vi "THzTimeAutoSave_PSD_TA.vi"(4 "ext. out":cluster{dbl[], dbl[], dbl[], dbl[], string[]}, 5 "Autosave Directory for Long-term Average Scan":path, 6 "y-axis":dbl[](array[numeric]), 7 "x-axis":sgl[](array[numeric]), 8 "String":string, 9 "SaveFile name":string) -> ()   [LabVIEW 2010]
uses:
  <vilib>/Utility/file.llb/Write To Spreadsheet File (DBL).vi
  <vilib>/Utility/file.llb/Write To Spreadsheet File (string).vi
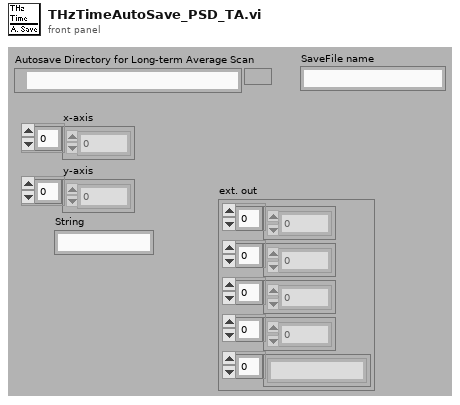
[diagram p1: front panel]
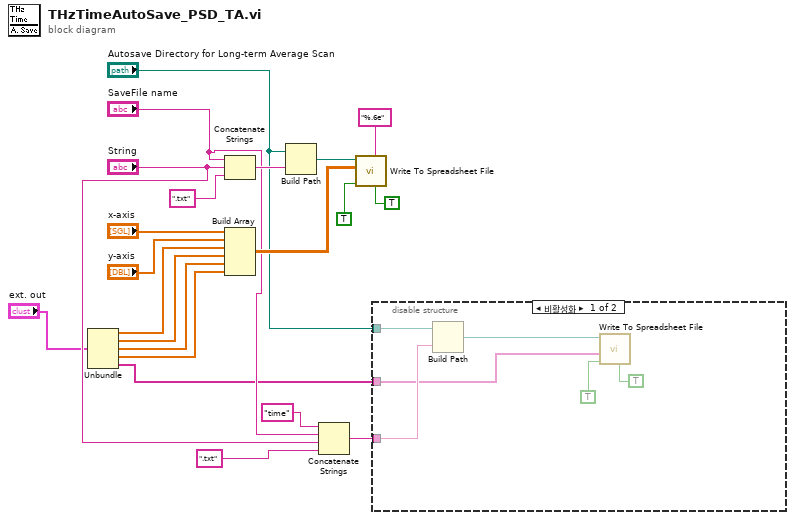
[diagram p0: block diagram]
diagram:
  n1 = Unbundle("ext. out") -> (w12:dbl[], w11:dbl[], w10:dbl[], w9:dbl[], w1:string[])
  n2 = Concatenate Strings("SaveFile name", "String", ".txt" ("string")) -> (w15:string)
  n3 = Build Array("x-axis", "y-axis", w12, w11, w10, w9) -> (w20:dbl[][])
  n4 = Build Path(base path="Autosave Directory for Long-term Average Scan", name or relative path=w15) -> (appended path=w21:path)
  n5 = Concatenate Strings("time" ("string"), "SaveFile name", "String", ".txt" ("string")) -> (w6:string)
  n6 = call-poly <vilib>:"Write To Spreadsheet File.vi"("transpose? (no:F)"=TRUE ("transpose?\n(no:F)"), "format (%.3f)"="%.6e", "append to file? (new file:F)"=TRUE ("transpose?\n(no:F)"), "2D data"=w20, "file path (dialog if empty)"=w21) -> ()  [unwired: 3 in, 1 out]
  n7 = disable-structure shown="비활성화" {
    disable-tunnel: w6 -> [w27 _]
    disable-tunnel: "Autosave Directory for Long-term Average Scan" -> [w23 _]
    disable-tunnel: w1 -> [w22 _]
    frame Disabled {
      n8 = Build Path(base path=w23, name or relative path=w27) -> (appended path=w24:path)
      n9 = call-poly <vilib>:"Write To Spreadsheet File.vi"("transpose? (no:F)"=TRUE ("transpose?\n(no:F)"), "append to file? (new file:F)"=TRUE ("transpose?\n(no:F)"), "1D data"=w22, "file path (dialog if empty)"=w24) -> ()  [unwired: 4 in, 1 out]
    }
    frame Enabled {
    }
  }
